vi "Set Byte Order.vi"(10 "byte order":T1, 11 "Transfer Configuration in":refnum<class "Transfer Configuration.lvclass">) -> (3 "Transfer Configuration out":refnum<class "Transfer Configuration.lvclass">)   [LabVIEW 2017, in "Data Sharing Framework Core.lvlib" / "Data Sharing Framework Engine.lvlib" / "Transfer Configuration.lvclass"]
uses:
  Transfer Configuration.lvclass
  Configuration/1.0.0/Public/Controls/DSF Byte Order.ctl
  Transfer Configuration.lvclass/Transfer Configuration.ctl
  Configuration/1.0.0/Data Sharing Framework Configuration.lvlib
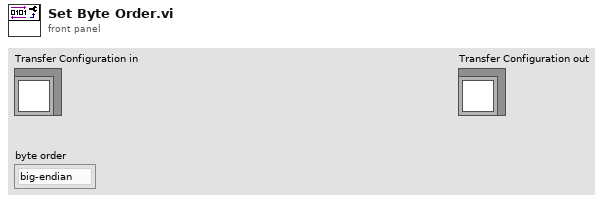
[diagram p1: front panel]
types:
  T1 = typedef "Data Sharing Framework Core.lvlib/Data Sharing Framework Configuration.lvlib/DSF Byte Order.ctl" = enum8{"big-endian", "little-endian"}
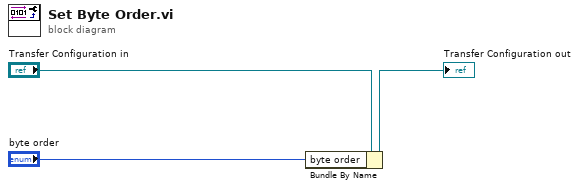
[diagram p0: block diagram]
diagram:
  n1 = Bundle By Name(cluster="Transfer Configuration in", "byte order"="byte order") -> (→"Transfer Configuration out":refnum<class "Transfer Configuration.lvclass">)
